vi "5Vote.vi"(10 "Input":bool=TRUE) -> (2 "vote5":bool)   [LabVIEW 2013, in "kevLib2011.lvlib"]
uses:
  kevLib2011.lvlib
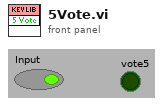
[diagram p1: front panel]
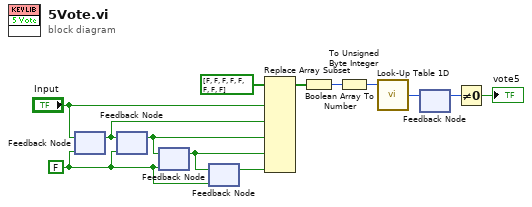
[diagram p0: block diagram]
diagram:
  w12 = FALSE ("Input")
  n1 = feedback-in #1("Input") -> ()
  n2 = feedback #1(w12) -> (w6:bool)
  n3 = feedback-in #2(w6) -> ()
  n4 = feedback #2(w12) -> (w5:bool)
  n5 = feedback-in #3(w5) -> ()
  n6 = feedback #3(w12) -> (w4:bool)
  n7 = feedback-in #4(w4) -> ()
  n8 = feedback #4(w12) -> (w3:bool)
  n9 = Replace Array Subset(array=bool[] [FALSE, FALSE, FALSE, FALSE, FALSE, FALSE, FALSE, FALSE], new element #1="Input", new element #2=w6, new element #3=w5, new element #4=w4, new element #5=w3) -> (w1:bool[])  [unwired: 5 in]
  n10 = Boolean Array To Number(Boolean array=w1) -> (number=w9:u8)
  n11 = To Unsigned Byte Integer(number=w9) -> (unsigned 8bit integer=w8:u8)
  n12 = call "Look-Up Table 1D"("address"=w8) -> ("data out"=w11:u8)  [unwired: 8 in]
  n13 = feedback-in #5(w11) -> ()
  n14 = feedback #5() -> (w10:u8)  [unwired: 1 out]
  n15 = Not Equal To 0?(x=w10) -> (x != 0?=→"vote5":bool)
